vi "test.vi"   [LabVIEW 2016]
uses:
  Classes/Controller/Motion/A3200 Folder/A3200.lvclass
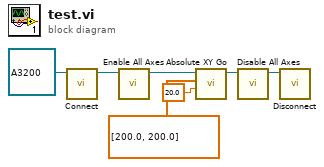
[diagram p0: block diagram]
diagram:
  n1 = call-dynamic "Connect.vi"("Gantry in"=refnum<class "A3200.lvclass"> refnum ("A3200.lvclass")) -> ("Gantry out"=w6:refnum<class "A3200.lvclass">)  [unwired: 9 in, 1 out]
  n2 = call-dynamic "Enable All Axes.vi"("A3200 in"=w6) -> ("A3200 out"=w5:refnum<class "A3200.lvclass">)  [unwired: 9 in, 1 out]
  n3 = call-dynamic "Absolute XY Go.vi"("Speed"=20.0, "XY"=dbl[] [200.0, 200.0], "Gantry in"=w5) -> ("Gantry out"=w4:refnum<class "A3200.lvclass">)  [unwired: 7 in, 1 out]
  n4 = call-dynamic "Disable All Axes.vi"("Gantry in"=w4) -> ("Gantry out"=w3:refnum<class "A3200.lvclass">)  [unwired: 9 in, 1 out]
  n5 = call-dynamic "Disconnect.vi"("Gantry in"=w3) -> ()  [unwired: 9 in, 1 out]
